vi "Add Connection.vi"(8 "error in (no error)":errorcluster, 9 "channel 2":string, 10 "channel 1":string, 11 "SLSC Switch in":refnum<class "SLSC Switch.lvclass">) -> (0 "error out":errorcluster, 3 "SLSC Switch out":refnum<class "SLSC Switch.lvclass">)   [LabVIEW 2015, in "SLSC Switch.lvclass"]
uses:
  SLSC Switch.lvclass
  Controls/Connection.ctl
  SLSC Switch.lvclass/SLSC Switch.ctl
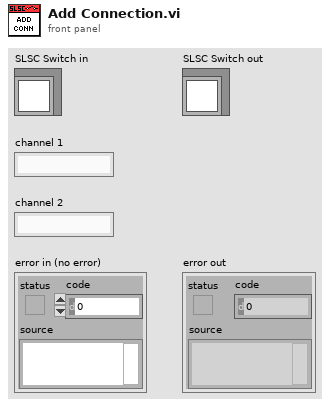
[diagram p1: front panel]
types:
  T1 = typedef "SLSC Switch.lvclass/Connection.ctl" = cluster{"channel 1":string, "channel 2":string}
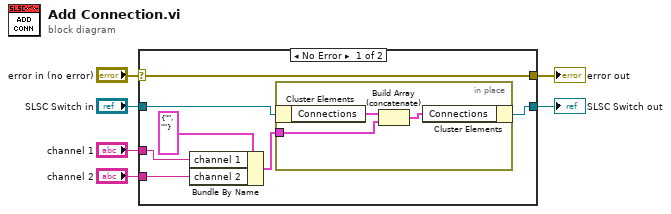
[diagram p0: block diagram]
diagram:
  n1 = case shown="No Error" "error in (no error)" {
    selector: "error in (no error)" -> [w13 w18]
    tunnel: [w13 w18] -> w5
    tunnel: [w11 w17] -> w3
    tunnel: "SLSC Switch in" -> [w12 w17]
    tunnel: "channel 1" -> [w9 _]
    tunnel: "channel 2" -> [w8 _]
    frame No Error {
      n2 = Bundle By Name(cluster=T1 {"channel 1"="", "channel 2"=""} ("connections"), "channel 1"=w9, "channel 2"=w8) -> (w7:T1)
      n3 = in-place {
        in-place-border: w7 -> [w15]
        n4 = in-place-cluster #1(w12) -> ("Connections"=w16:T1[])
        n5 = Build Array (concatenate)(w16, w15) -> (w14:T1[])
        n6 = in-place-cluster #1("Connections"=w14) -> (w11:refnum<class "SLSC Switch.lvclass">)
      }
    }
    frame Error {
    }
  }
  "error out" <- w5
  "SLSC Switch out" <- w3
